vi "create table parameters.vi"(10 "AI table":string[](array[string]), 11 "table name":string="XQ") -> (3 "create table parameters":string)   [LabVIEW 2019, in "PostgreSQL.lvlib"]
uses:
  PostgreSQL.lvlib
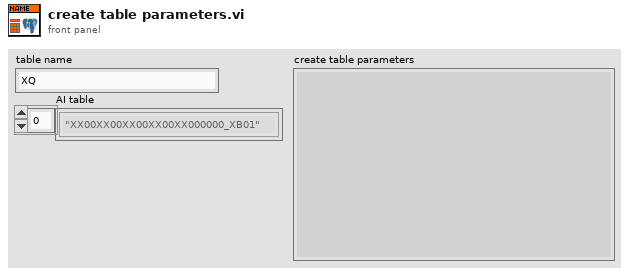
[diagram p1: front panel]
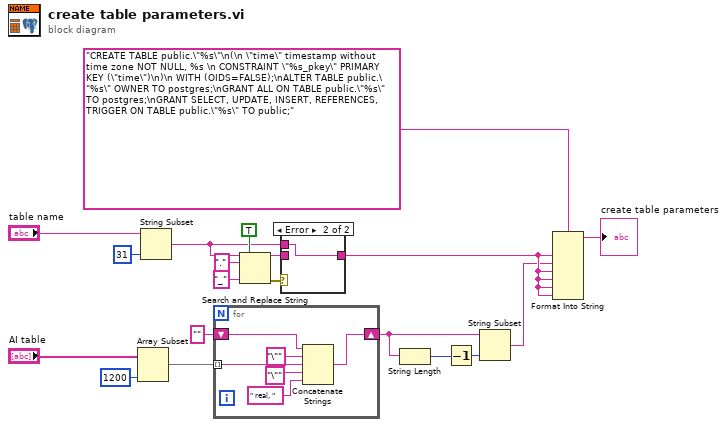
[diagram p0: block diagram]
diagram:
  n1 = Array Subset(array="AI table", length=1200) -> (w7:string[])  [unwired: 1 in]
  n2 = String Subset(string="table name", length (rest)=31 ("offset (0)")) -> (substring=w13:string)  [unwired: 1 in]
  n3 = for {
    tunnel: w7 -> [w23] mode=indexing
    shift-right: [w20] -> w2
    shift-left: "" ("result string") -> [w21]
    n4 = Concatenate Strings(w21, "\"" ("string"), w23, "\"" ("string"), " real, ") -> (w20:string)
  }
  n5 = Search and Replace String(replace all?=TRUE ("replace all? (F)"), input string=w13, search string=".", replace string="_" ("replace string (\"\")")) -> (result string=w16:string, error out=w17:errorcluster)  [unwired: 4 in, 2 out]
  n6 = case shown="Error" w17 {
    tunnel: w16 -> [w26 _]
    tunnel: [w26 w27] -> w6
    tunnel: w13 -> [_ w27]
    frame No Error {
    }
    frame Error {
    }
  }
  n7 = String Length(string=w2) -> (length=w1:i32)
  n8 = Decrement(x=w1) -> (x-1=w15:i32)
  n9 = String Subset(string=w2, length (rest)=w15) -> (substring=w5:string)  [unwired: 1 in]
  n10 = Format Into String(format string="CREATE TABLE public.\"%s\"\n(\n \"time\" timestamp without time zone NOT NULL, %s \n CONSTRAINT \"%s_pkey\" PRIMARY KEY (\"time\")\n)\n WITH (OIDS=FALSE);\nALTER TABLE public.\"%s\" OWNER TO postgres;\nGRANT ALL ON TABLE public.\"%s\" TO postgres;\nGRANT SELECT, UPDATE, INSERT, REFERENCES, TRIGGER ON TABLE public.\"%s\" TO public;", w6, w5, w6, w6, w6, w6) -> (resulting string=→"create table parameters":string)  [unwired: 2 in, 1 out]
